vi "Sistema_Aquisicao_queued.vi"() -> ()   [LabVIEW 2018]
uses:
  Global_Telescopio.vi
panel:
  out "respQ":refnum<queue>
  out "cmdQ":refnum<queue>
  out "error out":errorcluster
  out "ultimo valor 2":dbl format="%#_9g"
  out "ultimo valor":dbl format="%#_9g"
  out "ultimo comando":dbl
  in  "Case Constant\n(See Context Help)":bool=TRUE
  out "O Recebido":bool
  out "TimeoutAq":u32
  out "concatenated string":string
  out "Maq Satus":i32
  out "TX":string
  out "Data rx Aquisição":string
  # "2"
  # "R -->Registra Centragem\nS -->Status\nO -->OffSet\nF ---> Foco"
  # "3"
  # "4"
  # "5"
  # "!"
  # "!"
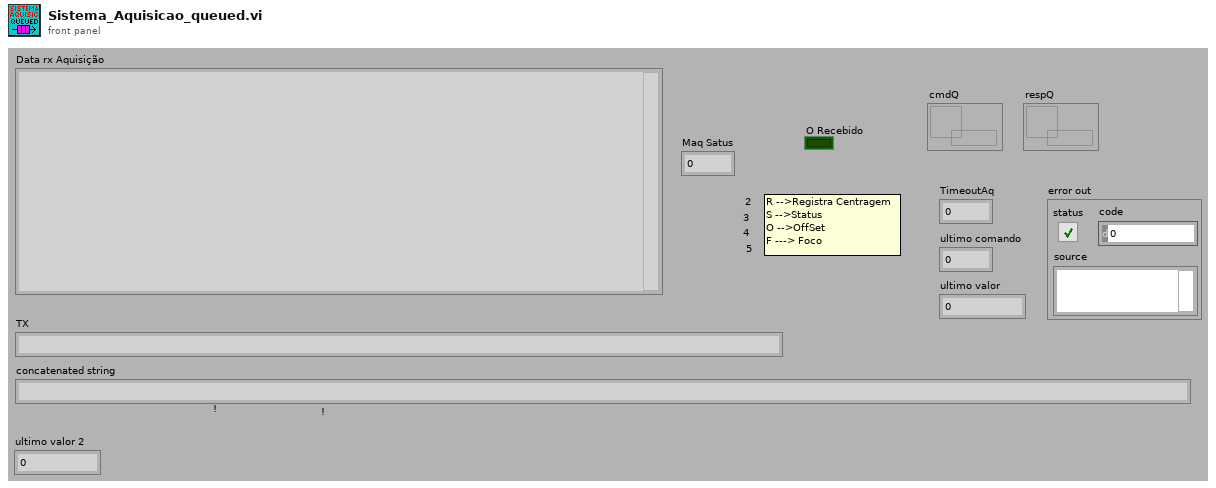
[diagram p1: front panel]
types:
  T1 = enum16{"open", "open or create", "create or replace", "create"}
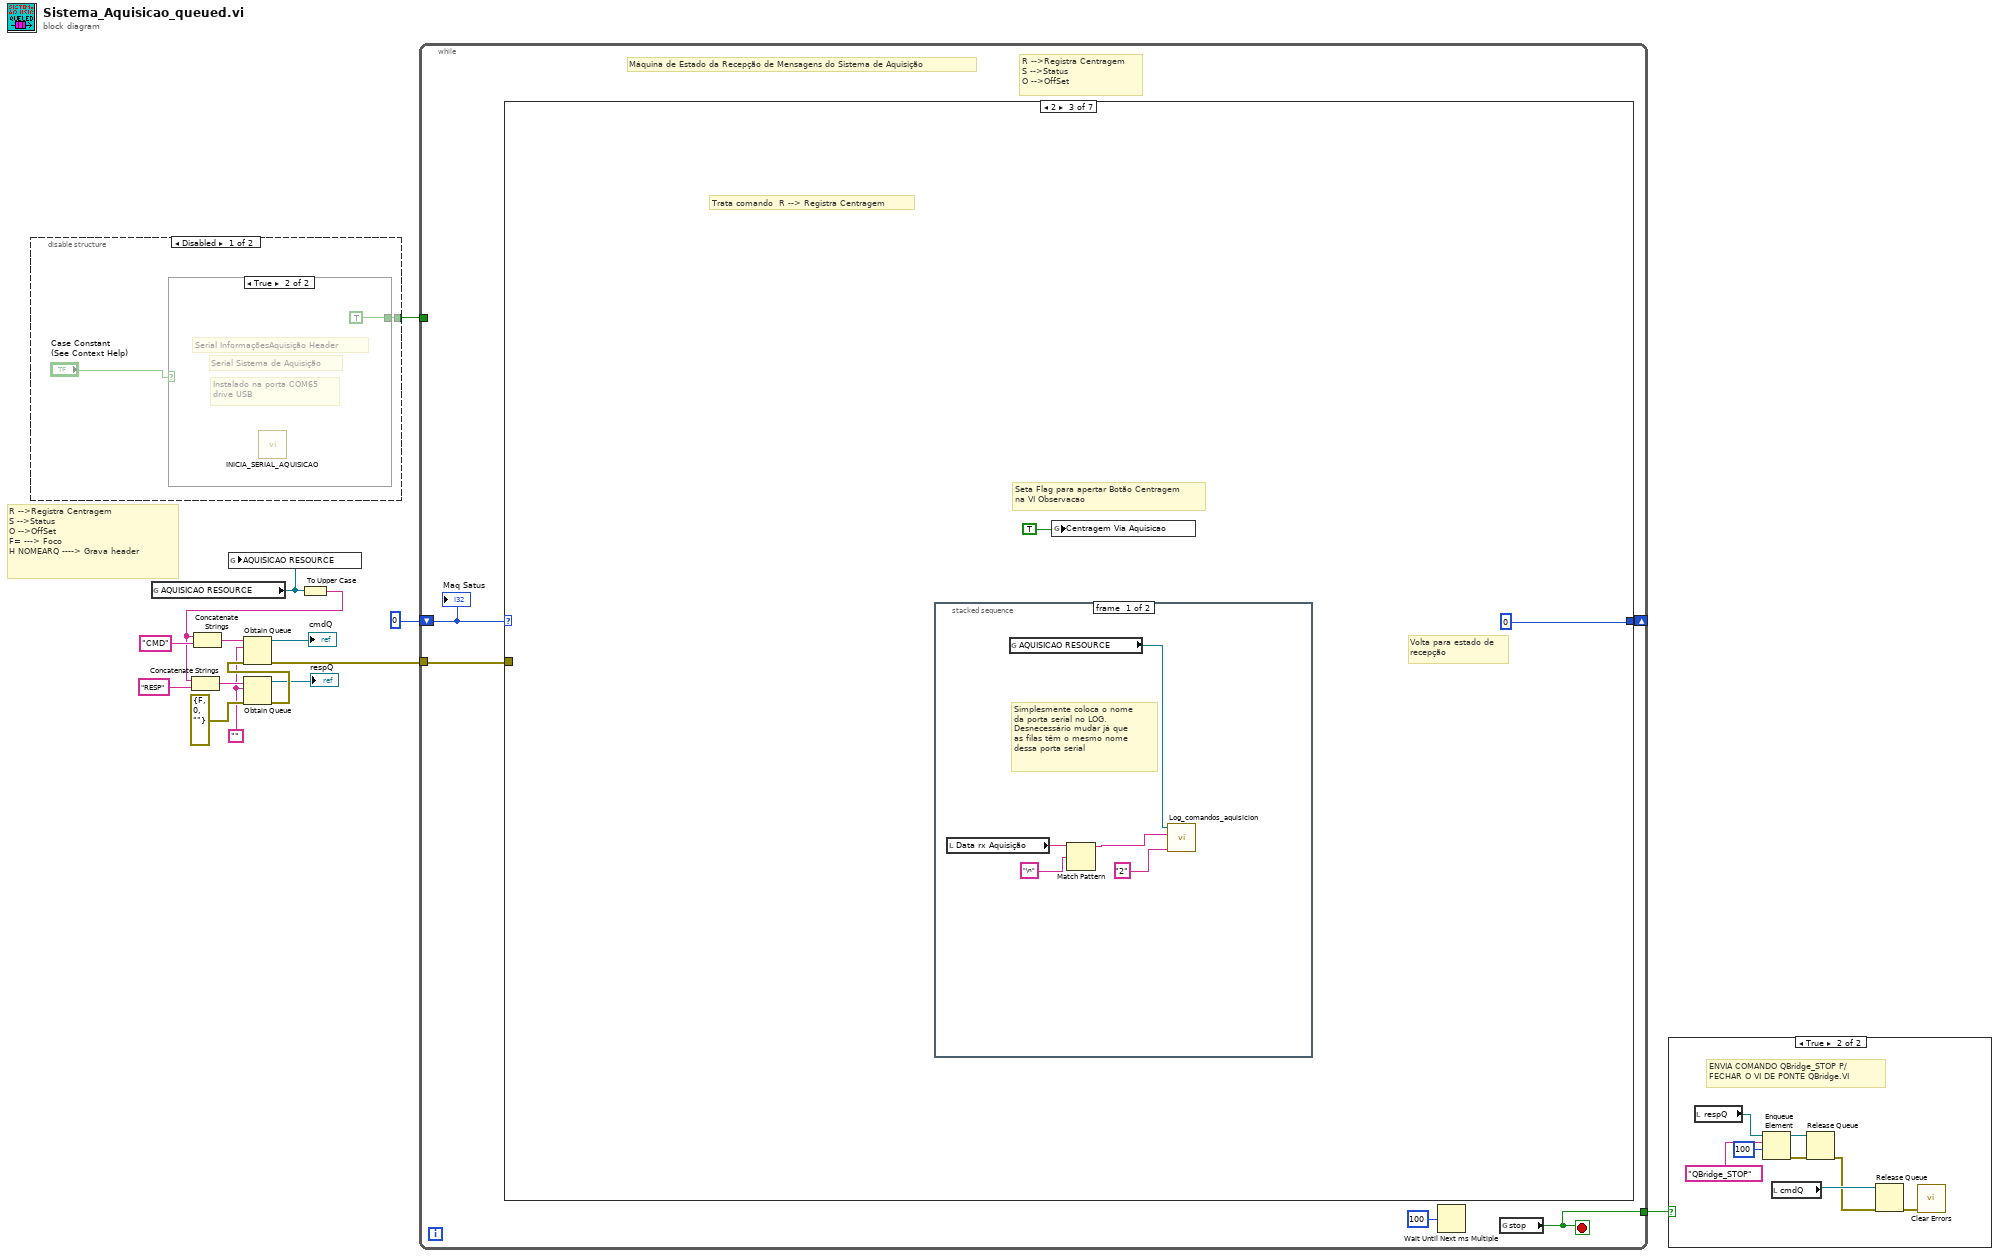
[diagram p0: block diagram]
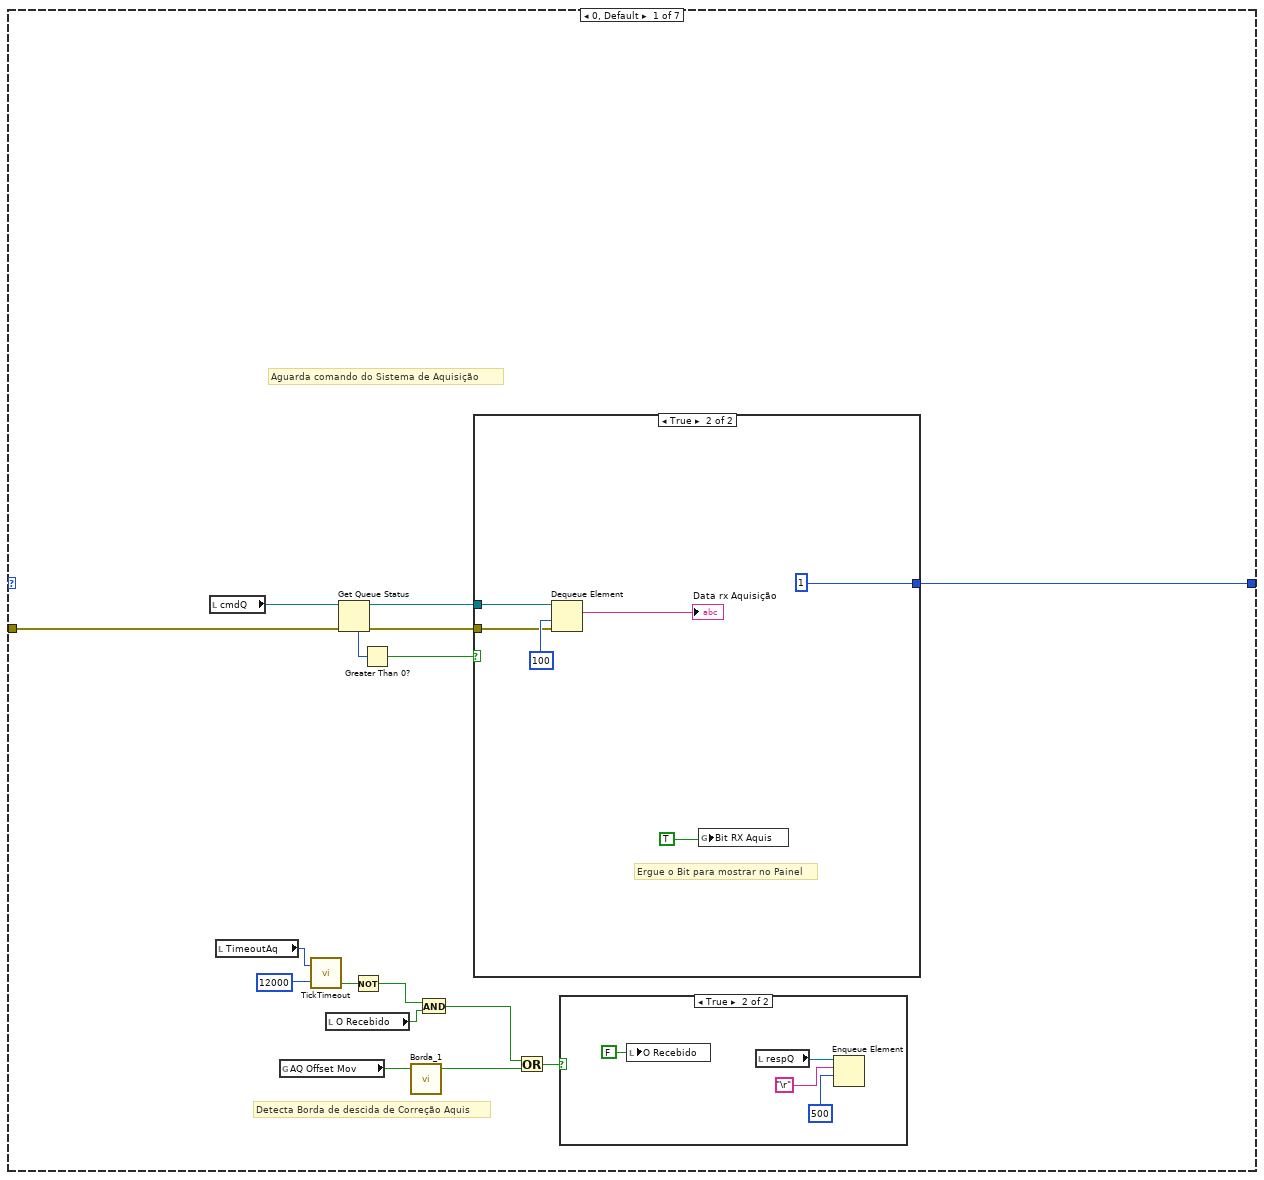
[diagram p5: hidden frame]
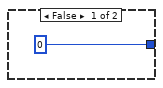
[diagram p7: hidden frame]
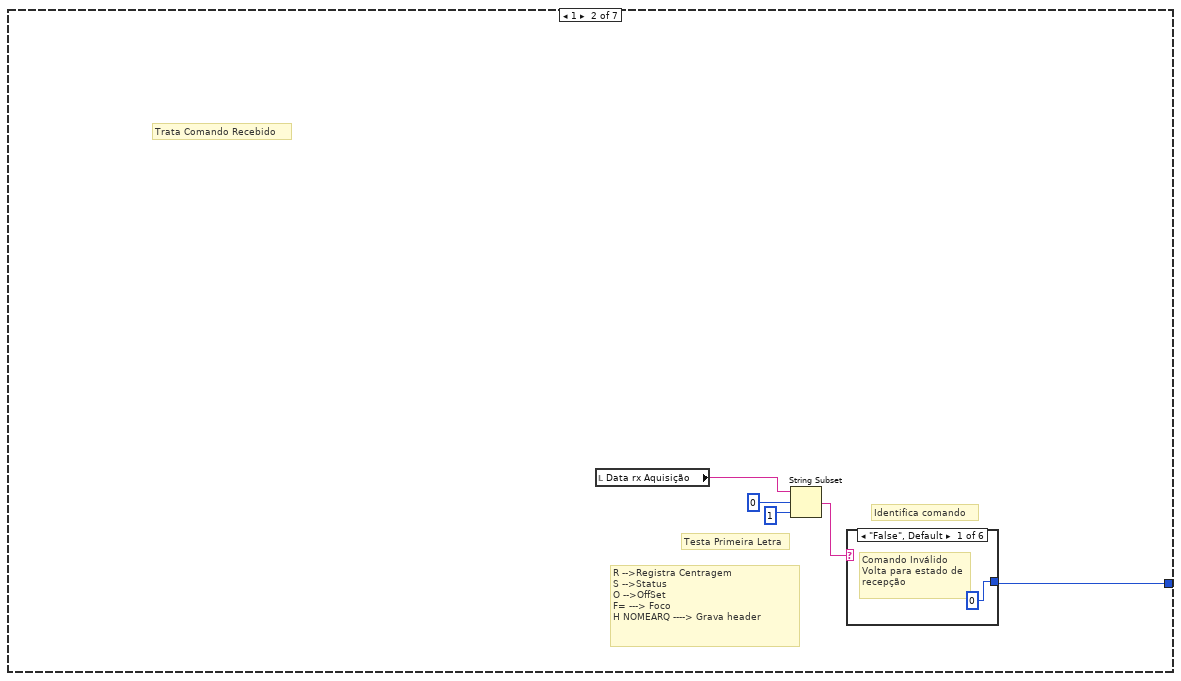
[diagram p8: hidden frame]
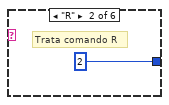
[diagram p9: hidden frame]
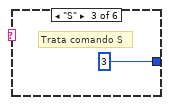
[diagram p10: hidden frame]
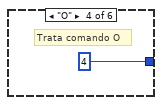
[diagram p11: hidden frame]
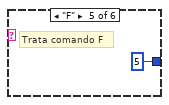
[diagram p12: hidden frame]
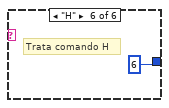
[diagram p13: hidden frame]
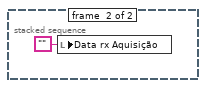
[diagram p14: hidden frame]
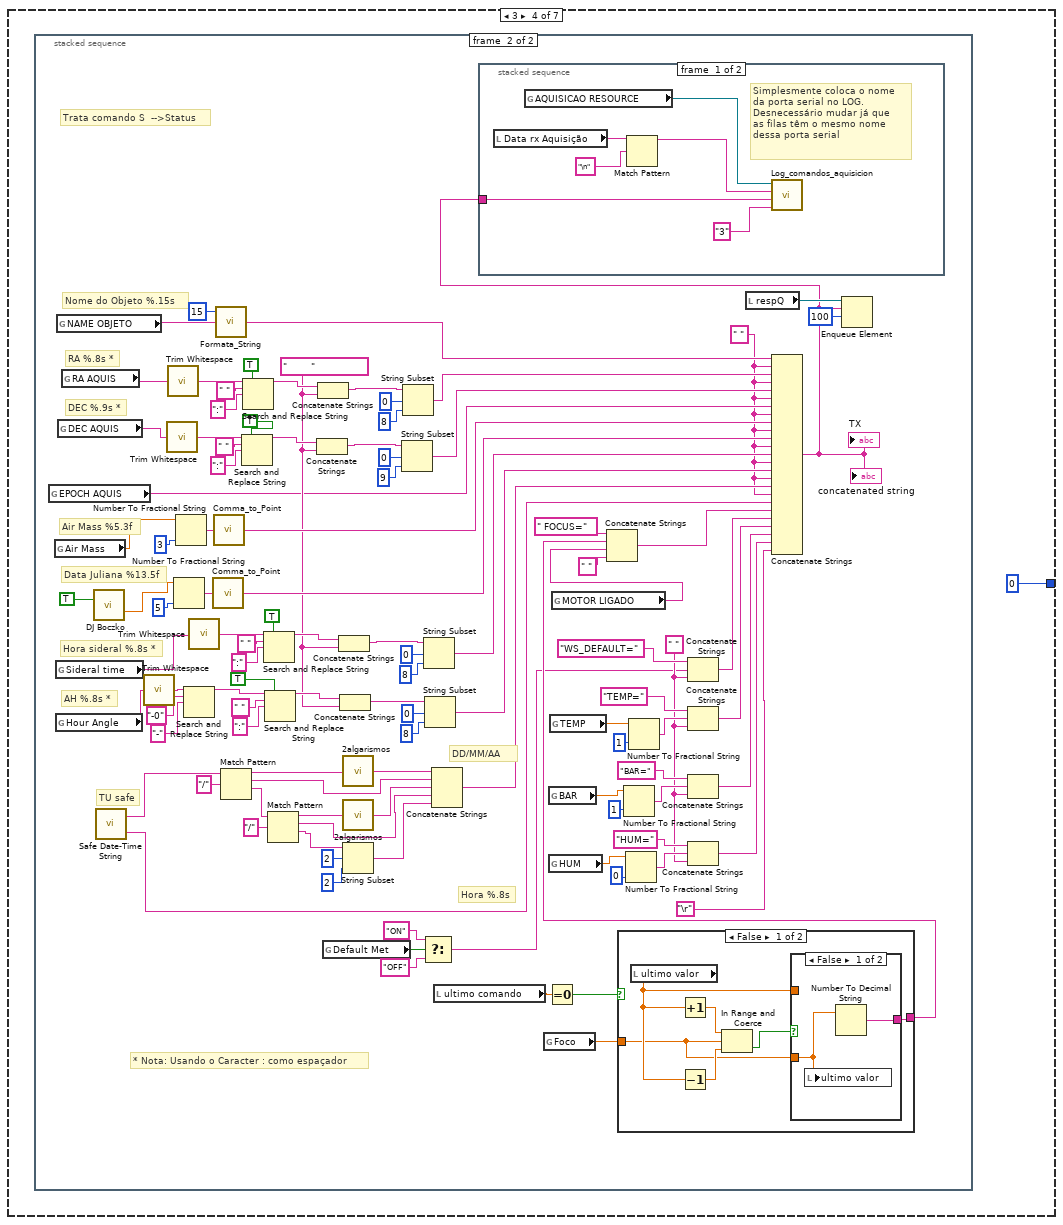
[diagram p15: hidden frame]
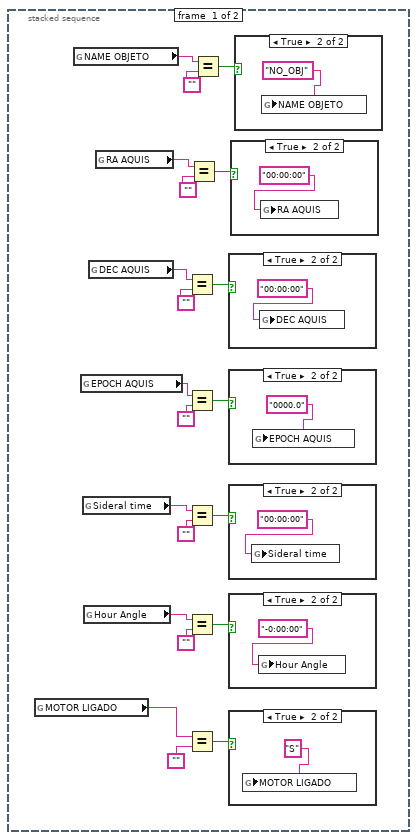
[diagram p16: hidden frame]
diagram:
  w5 = ""
  # "R -->Registra Centragem\nS -->Status\nO -->OffSet\nF= ---> Foco\nH NOMEARQ ----> Grava header"
  n1 = disable-structure shown="Disabled" {
    disable-tunnel: [w16 _] -> w14
    frame Disabled {
      n2 = case shown="True" "Case Constant\n(See Context Help)" {
        tunnel: [_ TRUE] -> w16
        frame False {
        }
        frame True {
          # "Instalado na porta COM65\ndrive USB"
          # "Serial Sistema de Aquisição"
          # "Serial InformaçõesAquisição Header"
          n3 = call "INICIA_SERIAL_AQUISICAO.vi"() -> ()  [unwired: 1 in]
        }
      }
    }
    frame Enabled {
    }
  }
  n4 = global read "Global_Telescopio.vi" "AQUISICAO RESOURCE"() -> (w3:refnum<visa-resource-name>)
  n5 = global write "Global_Telescopio.vi" "AQUISICAO RESOURCE"(w3) -> ()
  n6 = To Upper Case(1:w3) -> (0:w2:string)
  n7 = Concatenate Strings(w2, "RESP" ("string")) -> (w11:string)
  n8 = Concatenate Strings(w2, "CMD" ("string")) -> (w10:string)
  n9 = Obtain Queue(name (unnamed)=w11, element data type=w5, error in (no error)=errorcluster {"status"=FALSE, "code"=0, "source"=""}) -> (queue out=→"respQ":refnum<queue>, error out=w8:errorcluster)  [unwired: 2 in, 1 out]
  n10 = Obtain Queue(name (unnamed)=w10, element data type=w5, error in (no error)=w8) -> (queue out=→"cmdQ":refnum<queue>, error out=w4:errorcluster)  [unwired: 2 in, 1 out]
  n11 = while {
    shift-right: [w21] -> _
    shift-left: 0 -> [w22]
    tunnel: w14 -> [_]
    tunnel: w4 -> [w20]
    tunnel: [w19] -> w1
    stop <- w19 stop-if-true
    # "R -->Registra Centragem\nS -->Status\nO -->OffSet"
    # "Máquina de Estado da Recepção de Mensagens do Sistema de Aquisição"
    n12 = case shown="2" w22 {
      tunnel: [w39 w51 0 0 0 0 0] -> w21
      tunnel: w20 -> [w25 _ _ _ _ _ _]
      frame 0, Default {
        # "Detecta Borda de descida de Correção Aquis"
        # "Aguarda comando do Sistema de Aquisição"
        n13 = local read "cmdQ"() -> (w24:refnum<queue>)
        n14 = local read "TimeoutAq"() -> (w32:u32)
        n15 = global read "Global_Telescopio.vi" "AQ Offset Mov"() -> (w37:bool)
        n16 = call "TickTimeout.vi"("msInicial"=w32, "msTimeout"=u32 12000) -> ("Timeout"=w33:bool)  [unwired: 2 out]
        n17 = local read "O Recebido"() -> (w35:bool)
        n18 = Get Queue Status(queue=w24, error in (no error)=w25) -> (queue out=w26:refnum<queue>, error out=w27:errorcluster, # elements in queue=w29:i32)  [unwired: 1 in, 5 out]
        n19 = Not(x=w33) -> (.not. x?=w31:bool)
        n20 = Greater Than 0?(x=w29) -> (x > 0?=w28:bool)
        n21 = call "Borda_1.vi"("Entrada"=w37) -> ("Boolean"=w38:bool)  [unwired: 4 in]
        n22 = And(x=w31, y=w35) -> (x .and. y?=w30:bool)
        n23 = case shown="True" w28 {
          tunnel: [0 1] -> w39
          tunnel: w27 -> [_ w46]
          tunnel: w26 -> [_ w47]
          frame False {
          }
          frame True {
            # "Ergue o Bit para mostrar no Painel"
            n24 = Dequeue Element(queue=w47, timeout in ms (-1)=100, error in (no error)=w46) -> (element=→"Data rx Aquisição":string)  [unwired: 3 out]
            n25 = global write "Global_Telescopio.vi" "Bit RX Aquis"(TRUE) -> ()
          }
        }
        n26 = Or(x=w30, y=w38) -> (x .or. y?=w36:bool)
        n27 = case shown="True" w36 {
          frame False {
          }
          frame True {
            n28 = local write "O Recebido"(FALSE ("O Recebido")) -> ()
            n29 = local read "respQ"() -> (w42:refnum<queue>)
            n30 = Enqueue Element(queue=w42, element="\r", timeout in ms (-1)=500) -> ()  [unwired: 1 in, 3 out]
          }
        }
      }
      frame 1 {
        # "R -->Registra Centragem\nS -->Status\nO -->OffSet\nF= ---> Foco\nH NOMEARQ ----> Grava header"
        # "Testa Primeira Letra"
        # "Identifica comando"
        # "Trata Comando Recebido"
        n31 = local read "Data rx Aquisição"() -> (w52:string)
        n32 = String Subset(string=w52, offset (0)=0, length (rest)=1 ("length (rest)")) -> (substring=w55:string)
        n33 = case shown="\"False\", Default" w55 {
          tunnel: [0 2 3 4 5 6] -> w51
          frame "False", Default {
            # "Comando Inválido\nVolta para estado de\nrecepção"
          }
          frame "R" {
            # "Trata comando R"
          }
          frame "S" {
            # "Trata comando S"
          }
          frame "O" {
            # "Trata comando O"
          }
          frame "F" {
            # "Trata comando F"
          }
          frame "H" {
            # "Trata comando H"
          }
        }
      }
      frame 2 {
        # "Seta Flag para apertar Botão Centragem\nna VI Observacao"
        # "Trata comando  R --> Registra Centragem"
        # "Volta para estado de\nrecepção"
        n34 = stacked-sequence {
          frame #0 {
            # "Simplesmente coloca o nome\nda porta serial no LOG.\nDesnecessário mudar já que \nas filas têm o mesmo nome\ndessa porta serial"
            n35 = local read "Data rx Aquisição"() -> (w65:string)
            n36 = global read "Global_Telescopio.vi" "AQUISICAO RESOURCE"() -> (w68:refnum<visa-resource-name>)
            n37 = Match Pattern(string=w65, regular expression="\n") -> (before substring=w64:string)  [unwired: 1 in, 3 out]
            n38 = call "Log_comandos_aquisicion.vi"("Estado"="2", "string de comando"=w64, "Porta"=w68) -> ()  [unwired: 9 in]
          }
          frame #1 {
            n39 = local write "Data rx Aquisição"("") -> ()
          }
        }
        n40 = global write "Global_Telescopio.vi" "Centragem Via Aquisicao"(TRUE ("Comunicaçao ok guider")) -> ()
      }
      frame 3 {
        n41 = stacked-sequence {
          frame #0 {
            n42 = global read "Global_Telescopio.vi" "MOTOR LIGADO"() -> (w91:string)
            n43 = global read "Global_Telescopio.vi" "NAME OBJETO"() -> (w72:string)
            n44 = global read "Global_Telescopio.vi" "EPOCH AQUIS"() -> (w81:string)
            n45 = global read "Global_Telescopio.vi" "Sideral time"() -> (w83:string)
            n46 = global read "Global_Telescopio.vi" "Hour Angle"() -> (w88:string)
            n47 = global read "Global_Telescopio.vi" "DEC AQUIS"() -> (w79:string)
            n48 = global read "Global_Telescopio.vi" "RA AQUIS"() -> (w76:string)
            n49 = Equal?(x=w79, y="") -> (x = y?=w78:bool)
            n50 = Equal?(x=w81, y="") -> (x = y?=w80:bool)
            n51 = Equal?(x=w83, y="") -> (x = y?=w82:bool)
            n52 = Equal?(x=w88, y="") -> (x = y?=w84:bool)
            n53 = Equal?(x=w91, y="") -> (x = y?=w90:bool)
            n54 = Equal?(x=w76, y="") -> (x = y?=w74:bool)
            n55 = Equal?(x=w72, y="") -> (x = y?=w73:bool)
            n56 = case shown="True" w78 {
              frame False {
              }
              frame True {
                n57 = global write "Global_Telescopio.vi" "DEC AQUIS"("00:00:00" ("NAME OBJETO")) -> ()
              }
            }
            n58 = case shown="True" w80 {
              frame False {
              }
              frame True {
                n59 = global write "Global_Telescopio.vi" "EPOCH AQUIS"("0000.0" ("NAME OBJETO")) -> ()
              }
            }
            n60 = case shown="True" w82 {
              frame False {
              }
              frame True {
                n61 = global write "Global_Telescopio.vi" "Sideral time"("00:00:00" ("NAME OBJETO")) -> ()
              }
            }
            n62 = case shown="True" w84 {
              frame False {
              }
              frame True {
                n63 = global write "Global_Telescopio.vi" "Hour Angle"("-0:00:00" ("NAME OBJETO")) -> ()
              }
            }
            n64 = case shown="True" w90 {
              frame False {
              }
              frame True {
                n65 = global write "Global_Telescopio.vi" "MOTOR LIGADO"("S") -> ()
              }
            }
            n66 = case shown="True" w74 {
              frame False {
              }
              frame True {
                n67 = global write "Global_Telescopio.vi" "RA AQUIS"("00:00:00" ("NAME OBJETO")) -> ()
              }
            }
            n68 = case shown="True" w73 {
              frame False {
              }
              frame True {
                n69 = global write "Global_Telescopio.vi" "NAME OBJETO"("NO_OBJ" ("NAME OBJETO")) -> ()
              }
            }
          }
          frame #1 {
            w113 = " " ("string")
            w163 = "        " ("string")
            w121 = " "
            # "TU safe"
            # "* Nota: Usando o Caracter : como espaçador"
            # "Hora %.8s"
            # "DD/MM/AA"
            # "AH %.8s *"
            # "Hora sideral %.8s *"
            # "Data Juliana %13.5f"
            # "Air Mass %5.3f"
            # "DEC %.9s *"
            # "RA %.8s *"
            # "Nome do Objeto %.15s"
            # "Trata comando S  -->Status"
            n70 = global read "Global_Telescopio.vi" "EPOCH AQUIS"() -> (w136:string)
            n71 = global read "Global_Telescopio.vi" "Air Mass"() -> (w145:dbl)
            n72 = global read "Global_Telescopio.vi" "Sideral time"() -> (w172:string)
            n73 = global read "Global_Telescopio.vi" "Hour Angle"() -> (w137:string)
            n74 = global read "Global_Telescopio.vi" "NAME OBJETO"() -> (w144:string)
            n75 = global read "Global_Telescopio.vi" "DEC AQUIS"() -> (w189:string)
            n76 = global read "Global_Telescopio.vi" "RA AQUIS"() -> (w204:string)
            n77 = call "DJ Boczko.vi"("TRUE = Hora Local\nFALSE = UT"=TRUE ("TRUE = Hora Local\nFALSE = UT")) -> ("Dia Juliano"=w182:dbl)  [unwired: 6 in, 8 out]
            n78 = call "Safe Date-Time String.vi"() -> ("Safe time string"=w100:string, "Safe date string"=w99:string)  [unwired: 3 in]
            n79 = call <vilib>:"Trim Whitespace.vi"("string"=w137) -> ("trimmed string"=w138:string)  [unwired: 1 in]
            n80 = call <vilib>:"Trim Whitespace.vi"("string"=w189) -> ("trimmed string"=w192:string)  [unwired: 1 in]
            n81 = call <vilib>:"Trim Whitespace.vi"("string"=w204) -> ("trimmed string"=w203:string)  [unwired: 1 in]
            n82 = Number To Fractional String(number=w182, precision (6)=i16 5) -> (F-format string=w181:string)  [unwired: 2 in]
            n83 = Number To Fractional String(number=w145, precision (6)=i16 3) -> (F-format string=w185:string)  [unwired: 2 in]
            n84 = Search and Replace String(input string=w138, search string="-0", replace string="-" ("replace string (\"\")")) -> (result string=w139:string)  [unwired: 5 in, 3 out]
            n85 = call <vilib>:"Trim Whitespace.vi"("string"=w172) -> ("trimmed string"=w175:string)  [unwired: 1 in]
            n86 = call "Comma_to_Point.vi"("Lat_A"=w181) -> ("Saída"=w180:string)
            n87 = call "Comma_to_Point.vi"("Lat_A"=w185) -> ("Saída"=w184:string)
            n88 = call "Formata_String.vi"("entrada"=w144, "Num de Caracteres"=15) -> ("saida"=w142:string)  [unwired: 3 in]
            n89 = Match Pattern(string=w99, regular expression="/") -> (before substring=w158:string, match substring=w152:string, after substring=w159:string)  [unwired: 1 in, 1 out]
            n90 = Search and Replace String(replace all?=TRUE ("replace all? (F)"), input string=w192, search string=" ", replace string=":" ("replace string (\"\")")) -> (result string=w195:string)  [unwired: 4 in, 3 out]
            n91 = Search and Replace String(replace all?=TRUE ("replace all? (F)"), input string=w203, search string=" ", replace string=":" ("replace string (\"\")")) -> (result string=w199:string)  [unwired: 4 in, 3 out]
            n92 = Search and Replace String(replace all?=TRUE ("replace all? (F)"), input string=w175, search string=" ", replace string=":" ("replace string (\"\")")) -> (result string=w178:string)  [unwired: 4 in, 3 out]
            n93 = Search and Replace String(replace all?=TRUE ("replace all? (F)"), input string=w139, search string=" ", replace string=":" ("replace string (\"\")")) -> (result string=w165:string)  [unwired: 4 in, 3 out]
            n94 = Match Pattern(string=w159, regular expression="/") -> (before substring=w157:string, match substring=w150:string, after substring=w156:string)  [unwired: 1 in, 1 out]
            n95 = Concatenate Strings(w195, w163) -> (w196:string)
            n96 = Concatenate Strings(w199, w163) -> (w198:string)
            n97 = global read "Global_Telescopio.vi" "Default Met"() -> (w104:bool)
            n98 = Concatenate Strings(w178, w163) -> (w179:string)
            n99 = Concatenate Strings(w165, w163) -> (w164:string)
            n100 = call "2algarismos.vi"("entrada"=w158) -> ("saida"=w153:string)
            n101 = call "2algarismos.vi"("entrada"=w157) -> ("saida"=w151:string)
            n102 = String Subset(string=w156, offset (0)=2, length (rest)=2 ("length (rest)")) -> (substring=w149:string)
            n103 = String Subset(string=w196, offset (0)=0, length (rest)=9 ("length (rest)")) -> (substring=w188:string)
            n104 = String Subset(string=w198, offset (0)=0, length (rest)=8 ("length (rest)")) -> (substring=w197:string)
            n105 = Select(t="ON", s=w104, f="OFF") -> (s? t:f=w101:string)
            n106 = String Subset(string=w179, offset (0)=0, length (rest)=8 ("length (rest)")) -> (substring=w170:string)
            n107 = String Subset(string=w164, offset (0)=0, length (rest)=8 ("length (rest)")) -> (substring=w162:string)
            n108 = Concatenate Strings(w153, w152, w151, w150, w149) -> (w148:string)
            n109 = local read "ultimo comando"() -> (w135:dbl)
            n110 = global read "Global_Telescopio.vi" "Foco"() -> (w130:dbl)
            n111 = Equal To 0?(x=w135) -> (x = 0?=w134:bool)
            n112 = global read "Global_Telescopio.vi" "BAR"() -> (w123:dbl)
            n113 = global read "Global_Telescopio.vi" "HUM"() -> (w122:dbl)
            n114 = global read "Global_Telescopio.vi" "TEMP"() -> (w127:dbl)
            n115 = global read "Global_Telescopio.vi" "MOTOR LIGADO"() -> (w129:string)
            n116 = case shown="False" w134 {
              tunnel: [w215 w225] -> w133
              tunnel: w130 -> [w214 w224]
              frame False {
                n117 = local read "ultimo valor"() -> (w216:dbl)
                n118 = Increment(x=w216) -> (x+1=w218:dbl)
                n119 = Decrement(x=w216) -> (x-1=w217:dbl)
                n120 = In Range and Coerce(upper limit=w218, x=w214, lower limit=w217) -> (In Range?=w219:bool)  [unwired: 1 out]
                n121 = case shown="False" w219 {
                  tunnel: w216 -> [_ w223]
                  tunnel: [w221 w222] -> w215
                  tunnel: w214 -> [w220 _]
                  frame False {
                    n122 = local write "ultimo valor"(w220) -> ()
                    n123 = Number To Decimal String(number=w220) -> (decimal integer string=w221:string)  [unwired: 1 in]
                  }
                  frame True {
                    n124 = Number To Decimal String(number=w223) -> (decimal integer string=w222:string)  [unwired: 1 in]
                  }
                }
              }
              frame True {
                n125 = Number To Decimal String(number=w224) -> (decimal integer string=w225:string)  [unwired: 1 in]
                "ultimo valor" <- w224
              }
            }
            n126 = Concatenate Strings(" FOCUS=" ("string"), w133, w129, " " ("string")) -> (w131:string)
            n127 = Number To Fractional String(number=w123, precision (6)=i16 1) -> (F-format string=w115:string)  [unwired: 2 in]
            n128 = Number To Fractional String(number=w122, precision (6)=i16 0) -> (F-format string=w114:string)  [unwired: 2 in]
            n129 = Number To Fractional String(number=w127, precision (6)=i16 1) -> (F-format string=w117:string)  [unwired: 2 in]
            n130 = Concatenate Strings("WS_DEFAULT=" ("string"), w101, w113) -> (w112:string)
            n131 = Concatenate Strings("TEMP=" ("string"), w117, w113) -> (w111:string)
            n132 = Concatenate Strings("BAR=" ("string"), w115, w113) -> (w110:string)
            n133 = Concatenate Strings("HUM=" ("string"), w114, w113) -> (w109:string)
            n134 = local read "respQ"() -> (w107:refnum<queue>)
            n135 = Concatenate Strings(w142, w121, w197, w121, w188, w121, w136, w121, w184, w121, w180, w121, w170, w121, w162, w121, w148, w121, w100, w131, w112, w111, w110, w109, "\r") -> (w106:string)
            "TX" <- w106
            "concatenated string" <- w106
            n136 = stacked-sequence {
              tunnel: w106 -> [w210 _]
              frame #0 {
                # "Simplesmente coloca o nome\nda porta serial no LOG.\nDesnecessário mudar já que \nas filas têm o mesmo nome\ndessa porta serial"
                n137 = local read "Data rx Aquisição"() -> (w209:string)
                n138 = global read "Global_Telescopio.vi" "AQUISICAO RESOURCE"() -> (w212:refnum<visa-resource-name>)
                n139 = Match Pattern(string=w209, regular expression="\n") -> (before substring=w207:string)  [unwired: 1 in, 3 out]
                n140 = call "Log_comandos_aquisicion.vi"("Estado"="3", "string de Resposta"=w210, "string de comando"=w207, "Porta"=w212) -> ()  [unwired: 8 in]
              }
              frame #1 {
                n141 = local write "Data rx Aquisição"("") -> ()
              }
            }
            n142 = Enqueue Element(queue=w107, element=w106, timeout in ms (-1)=100) -> ()  [unwired: 1 in, 3 out]
          }
        }
      }
      frame 4 {
        # "Trata comando O  -->OffSet"
        n143 = local read "Data rx Aquisição"() -> (w228:string)
        n144 = String Subset(string=w228, offset (0)=2, length (rest)=1 ("length (rest)")) -> (substring=w237:string)
        n145 = String Subset(string=w228, offset (0)=3, length (rest)=4 ("length (rest)")) -> (substring=w244:string)
        n146 = String Subset(string=w228, offset (0)=8, length (rest)=1 ("length (rest)")) -> (substring=w236:string)
        n147 = String Subset(string=w228, offset (0)=1, length (rest)=1 ("length (rest)")) -> (substring=w230:string)
        n148 = String Subset(string=w228, offset (0)=9, length (rest)=4 ("length (rest)")) -> (substring=w243:string)
        n149 = Fract/Exp String To Number(use system decimal point (T)=FALSE, string=w244) -> (number=w233:dbl)  [unwired: 2 in, 1 out]
        n150 = Fract/Exp String To Number(use system decimal point (T)=FALSE, string=w243) -> (number=w231:dbl)  [unwired: 2 in, 1 out]
        n151 = case shown="\"N\"" w237 {
          tunnel: [0.0 ("PreciseOffsetDEC 2") 1.0 ("PreciseOffsetDEC 2") -1.0 ("PreciseOffsetDEC 2")] -> w234
          frame " ", Default {
          }
          frame "N" {
          }
          frame "S" {
          }
        }
        n152 = case shown="\"E\"" w236 {
          tunnel: [0.0 ("PreciseOffsetDEC 2") 1.0 ("PreciseOffsetDEC 2") -1.0 ("PreciseOffsetDEC 2")] -> w232
          frame " ", Default {
          }
          frame "W" {
          }
          frame "E" {
          }
        }
        n153 = call "Salva_comando_Apend.vi"("String"=w228, "file name p/ exell"="C:\\TCS\\LOG\\Comando_O_Aquisicao.txt") -> ()  [unwired: 4 in]
        n154 = Multiply(x=w234, y=w232) -> (x*y=w238:dbl)
        n155 = Equal To 0?(x=w238) -> (x = 0?=w235:bool)
        n156 = case shown="True" w235 {
          tunnel: w234 -> [w271 _]
          tunnel: w233 -> [w270 _]
          tunnel: w232 -> [w269 _]
          tunnel: w231 -> [w268 _]
          tunnel: w230 -> [w266 _]
          tunnel: [TRUE ("Correção Aquis") FALSE ("Correção Aquis")] -> w229
          tunnel: ["" ""] -> w226
          frame False {
            n157 = Multiply(x=w271, y=w270) -> (x*y=w263:dbl)
            n158 = Multiply(x=w269, y=w268) -> (x*y=w267:dbl)
            n159 = case shown="\"1\"" w266 {
              tunnel: [1.0 ("PreciseOffsetDEC 2") w273] -> w265
              frame "0", Default {
              }
              frame "1" {
                n160 = global read "Global_Telescopio.vi" "delta_now"() -> (w274:dbl)
                n161 = Cosine(x=w274) -> (cos(x)=w275:dbl)
                n162 = Absolute Value(x=w275) -> (abs(x)=w273:dbl)
              }
            }
            n163 = Divide(x=w267, y=w265) -> (x/y=w264:dbl)
            n164 = global write "Global_Telescopio.vi" "aquis_asc"(w264) -> ()
            n165 = global write "Global_Telescopio.vi" "aquis_dec"(w263) -> ()
            n166 = call "TickTimeout.vi"() -> ("msTick"=→"TimeoutAq":u32)  [unwired: 2 in, 2 out]
          }
          frame True {
          }
        }
        "O Recebido" <- w229
        n167 = stacked-sequence {
          tunnel: w226 -> [_ w259]
          frame #0 {
            n168 = local read "Data rx Aquisição"() -> (w255:string)
            n169 = global read "Global_Telescopio.vi" "AQUISICAO RESOURCE"() -> (w258:refnum<visa-resource-name>)
            n170 = Match Pattern(string=w255, regular expression="\n") -> (before substring=w254:string)  [unwired: 1 in, 3 out]
            n171 = call "Log_comandos_aquisicion.vi"("Estado"="4", "string de comando"=w254, "Porta"=w258) -> ()  [unwired: 9 in]
          }
          frame #1 {
            n172 = local write "Data rx Aquisição"(w259) -> ()
          }
        }
        n173 = global write "Global_Telescopio.vi" "Correção Aquis"(w229) -> ()
      }
      frame 5 {
        # "Trata comando F ---> Trata o comando de foco vindo do computador de aquisição"
        n174 = local read "Data rx Aquisição"() -> (w292:string)
        n175 = Match Pattern(string=w292, regular expression="=") -> (after substring=w290:string)  [unwired: 1 in, 3 out]
        n176 = Fract/Exp String To Number(string=w290) -> (number=w286:dbl)  [unwired: 3 in, 1 out]
        n177 = In Range and Coerce(upper limit=2012.0, x=w286, lower limit=1.0) -> (In Range?=w287:bool)  [unwired: 1 out]
        n178 = case shown="True" w287 {
          tunnel: w286 -> [_ w302]
          tunnel: ["" ""] -> w284
          frame False {
          }
          frame True {
            n179 = case shown="True" TRUE {
              tunnel: ["stop" ("Comando") "go" ("Comando")] -> w301
              frame False {
              }
              frame True {
                n180 = call "TX focus FOCO.vi"("Comando"="def", "Setpoint"=20.0) -> ()  [unwired: 11 in, 3 out]
              }
            }
            n181 = call "TX focus FOCO.vi"("Comando"=w301, "Setpoint"=w302) -> ()  [unwired: 11 in, 3 out]
            "ultimo comando" <- w302
          }
        }
        n182 = stacked-sequence {
          tunnel: w284 -> [_ w298]
          frame #0 {
            n183 = local read "Data rx Aquisição"() -> (w294:string)
            n184 = global read "Global_Telescopio.vi" "AQUISICAO RESOURCE"() -> (w297:refnum<visa-resource-name>)
            n185 = Match Pattern(string=w294, regular expression="\n") -> (before substring=w293:string)  [unwired: 1 in, 3 out]
            n186 = call "Log_comandos_aquisicion.vi"("Estado"="5", "string de comando"=w293, "Porta"=w297) -> ()  [unwired: 9 in]
          }
          frame #1 {
            n187 = local write "Data rx Aquisição"(w298) -> ()
          }
        }
      }
      frame 6 {
        w338 = " " ("string")
        w388 = "        " ("string")
        w346 = " "
        # "TU safe"
        # "ANTES DE INTRODUZIR FILAS\nESTA ESTRUTURA DISABLE JÁ\nESTAVA PRESENTE NO CÓDIGO"
        # "file name"
        # "* Nota: Usando o Caracter : como espaçador"
        # "Hora %.8s"
        # "DD/MM/AA"
        # "AH %.8s *"
        # "Hora sideral %.8s *"
        # "Data Juliana %13.5f"
        # "Air Mass %5.3f"
        # "DEC %.9s *"
        # "RA %.8s *"
        # "Nome do Objeto %.15s"
        # "Trata comando H NOMEARQ ---> Grava Header"
        n188 = global read "Global_Telescopio.vi" "EPOCH AQUIS"() -> (w361:string)
        n189 = global read "Global_Telescopio.vi" "Air Mass"() -> (w370:dbl)
        n190 = global read "Global_Telescopio.vi" "Sideral time"() -> (w397:string)
        n191 = global read "Global_Telescopio.vi" "Hour Angle"() -> (w362:string)
        n192 = global read "Global_Telescopio.vi" "NAME OBJETO"() -> (w369:string)
        n193 = global read "Global_Telescopio.vi" "DEC AQUIS"() -> (w414:string)
        n194 = global read "Global_Telescopio.vi" "RA AQUIS"() -> (w429:string)
        n195 = call "DJ Boczko.vi"("TRUE = Hora Local\nFALSE = UT"=TRUE ("TRUE = Hora Local\nFALSE = UT")) -> ("Dia Juliano"=w407:dbl)  [unwired: 6 in, 8 out]
        n196 = call "Safe Date-Time String.vi"() -> ("Safe time string"=w309:string, "Safe date string"=w308:string)  [unwired: 3 in]
        n197 = call <vilib>:"Trim Whitespace.vi"("string"=w362) -> ("trimmed string"=w363:string)  [unwired: 1 in]
        n198 = local read "Data rx Aquisição"() -> (w332:string)
        n199 = call <vilib>:"Trim Whitespace.vi"("string"=w414) -> ("trimmed string"=w417:string)  [unwired: 1 in]
        n200 = call <vilib>:"Trim Whitespace.vi"("string"=w429) -> ("trimmed string"=w428:string)  [unwired: 1 in]
        n201 = Number To Fractional String(number=w407, precision (6)=i16 5) -> (F-format string=w406:string)  [unwired: 2 in]
        n202 = Number To Fractional String(number=w370, precision (6)=i16 3) -> (F-format string=w410:string)  [unwired: 2 in]
        n203 = Search and Replace String(input string=w363, search string="-0", replace string="-" ("replace string (\"\")")) -> (result string=w364:string)  [unwired: 5 in, 3 out]
        n204 = call <vilib>:"Trim Whitespace.vi"("string"=w397) -> ("trimmed string"=w400:string)  [unwired: 1 in]
        n205 = Match Pattern(string=w332, regular expression="H ") -> (after substring=w317:string)  [unwired: 1 in, 3 out]
        n206 = call "Comma_to_Point.vi"("Lat_A"=w406) -> ("Saída"=w405:string)
        n207 = call "Comma_to_Point.vi"("Lat_A"=w410) -> ("Saída"=w409:string)
        n208 = call "Formata_String.vi"("entrada"=w369, "Num de Caracteres"=15) -> ("saida"=w367:string)  [unwired: 3 in]
        n209 = Match Pattern(string=w308, regular expression="/") -> (before substring=w383:string, match substring=w377:string, after substring=w384:string)  [unwired: 1 in, 1 out]
        n210 = global read "Global_Telescopio.vi" "Default Met"() -> (w313:bool)
        n211 = Search and Replace String(replace all?=TRUE ("replace all? (F)"), input string=w417, search string=" ", replace string=":" ("replace string (\"\")")) -> (result string=w420:string)  [unwired: 4 in, 3 out]
        n212 = Search and Replace String(replace all?=TRUE ("replace all? (F)"), input string=w428, search string=" ", replace string=":" ("replace string (\"\")")) -> (result string=w424:string)  [unwired: 4 in, 3 out]
        n213 = Search and Replace String(replace all?=TRUE ("replace all? (F)"), input string=w400, search string=" ", replace string=":" ("replace string (\"\")")) -> (result string=w403:string)  [unwired: 4 in, 3 out]
        n214 = Search and Replace String(replace all?=TRUE ("replace all? (F)"), input string=w364, search string=" ", replace string=":" ("replace string (\"\")")) -> (result string=w390:string)  [unwired: 4 in, 3 out]
        n215 = Match Pattern(string=w384, regular expression="/") -> (before substring=w382:string, match substring=w375:string, after substring=w381:string)  [unwired: 1 in, 1 out]
        n216 = Match Pattern(string=w317, regular expression="\r\n") -> (before substring=w315:string)  [unwired: 1 in, 3 out]
        n217 = Concatenate Strings(w420, w388) -> (w421:string)
        n218 = Concatenate Strings(w424, w388) -> (w423:string)
        n219 = Select(t="ON", s=w313, f="OFF") -> (s? t:f=w310:string)
        n220 = Concatenate Strings(w403, w388) -> (w404:string)
        n221 = Concatenate Strings(w390, w388) -> (w389:string)
        n222 = call "2algarismos.vi"("entrada"=w383) -> ("saida"=w378:string)
        n223 = call "2algarismos.vi"("entrada"=w382) -> ("saida"=w376:string)
        n224 = String Subset(string=w381, offset (0)=2, length (rest)=2 ("length (rest)")) -> (substring=w374:string)
        n225 = String Subset(string=w421, offset (0)=0, length (rest)=9 ("length (rest)")) -> (substring=w413:string)
        n226 = String Subset(string=w423, offset (0)=0, length (rest)=8 ("length (rest)")) -> (substring=w422:string)
        n227 = String Subset(string=w404, offset (0)=0, length (rest)=8 ("length (rest)")) -> (substring=w395:string)
        n228 = String Subset(string=w389, offset (0)=0, length (rest)=8 ("length (rest)")) -> (substring=w387:string)
        n229 = Concatenate Strings(w378, w377, w376, w375, w374) -> (w373:string)
        n230 = local read "ultimo comando"() -> (w360:dbl)
        n231 = global read "Global_Telescopio.vi" "Foco"() -> (w355:dbl)
        n232 = Equal To 0?(x=w360) -> (x = 0?=w359:bool)
        n233 = global read "Global_Telescopio.vi" "BAR"() -> (w348:dbl)
        n234 = global read "Global_Telescopio.vi" "HUM"() -> (w347:dbl)
        n235 = global read "Global_Telescopio.vi" "TEMP"() -> (w352:dbl)
        n236 = global read "Global_Telescopio.vi" "MOTOR LIGADO"() -> (w354:string)
        n237 = Concatenate Strings("C:\\TCS\\LOG\\HEADER\\" ("string"), w315, ".txt" ("string")) -> (w322:string)
        n238 = case shown="False" w359 {
          tunnel: [w436 w446] -> w358
          tunnel: w355 -> [w435 w445]
          frame False {
            n239 = local read "ultimo valor 2"() -> (w437:dbl)
            n240 = Increment(x=w437) -> (x+1=w439:dbl)
            n241 = Decrement(x=w437) -> (x-1=w438:dbl)
            n242 = In Range and Coerce(upper limit=w439, x=w435, lower limit=w438) -> (In Range?=w440:bool)  [unwired: 1 out]
            n243 = case shown="False" w440 {
              tunnel: w437 -> [_ w444]
              tunnel: [w442 w443] -> w436
              tunnel: w435 -> [w441 _]
              frame False {
                n244 = local write "ultimo valor 2"(w441) -> ()
                n245 = Number To Decimal String(number=w441) -> (decimal integer string=w442:string)  [unwired: 1 in]
              }
              frame True {
                n246 = Number To Decimal String(number=w444) -> (decimal integer string=w443:string)  [unwired: 1 in]
              }
            }
          }
          frame True {
            n247 = Number To Decimal String(number=w445) -> (decimal integer string=w446:string)  [unwired: 1 in]
            "ultimo valor 2" <- w445
          }
        }
        n248 = Concatenate Strings(" FOCUS=" ("string"), w358, w354, " " ("string")) -> (w356:string)
        n249 = Number To Fractional String(number=w348, precision (6)=i16 1) -> (F-format string=w340:string)  [unwired: 2 in]
        n250 = Number To Fractional String(number=w347, precision (6)=i16 0) -> (F-format string=w339:string)  [unwired: 2 in]
        n251 = Number To Fractional String(number=w352, precision (6)=i16 1) -> (F-format string=w342:string)  [unwired: 2 in]
        n252 = String To Path(string=w322) -> (path=w320:path)
        n253 = call <vilib>:"Open_Create_Replace File.vi"("function (open:0)"=T1."open or create", "file path"=w320) -> ("error out"=w327:errorcluster, "refnum"=w330:refnum<file>)  [unwired: 6 in, 2 out]
        n254 = Concatenate Strings("WS_DEFAULT=" ("string"), w310, w338) -> (w337:string)
        n255 = Concatenate Strings("TEMP=" ("string"), w342, w338) -> (w336:string)
        n256 = Concatenate Strings("BAR=" ("string"), w340, w338) -> (w335:string)
        n257 = Concatenate Strings("HUM=" ("string"), w339, w338) -> (w334:string)
        n258 = Set File Position(refnum=w330, from (0:start)=enum16{"start", "end", "current"}."end" ("pos mode (0:2)"), error in=w327) -> (refnum out=w324:refnum<file>, error out=w323:errorcluster)  [unwired: 1 in]
        n259 = Concatenate Strings(w367, w346, w422, w346, w413, w346, w361, w346, w409, w346, w405, w346, w395, w346, w387, w346, w373, w346, w309, w356, w337, w336, w335, w334, "\r") -> (w319:string)
        n260 = disable-structure shown="Disabled" {
          disable-tunnel: w319 -> [w433 _]
          frame Disabled {
            n261 = global read "Global_Telescopio.vi" "AQUISICAO RESOURCE"() -> (w434:refnum<visa-resource-name>)
            n262 = call "TX.vi"("tx_buf"=w433, "VISA resource name"=w434) -> ()  [unwired: 1 in, 3 out]
          }
          frame Enabled {
          }
        }
        n263 = Write to Text File(file (use dialog)=w324, text=w319, error in=w323) -> (refnum out=w329:refnum<file>, error out=w328:errorcluster)  [unwired: 1 in, 1 out]
        n264 = Close File(refnum=w329, error in=w328) -> (error out=→"error out":errorcluster)  [unwired: 1 out]
      }
    }
    n265 = Wait Until Next ms Multiple(millisecond multiple=u32 100) -> ()  [unwired: 1 out]
    n266 = global read "Global_Telescopio.vi" "stop"() -> (w19:bool)
    "Maq Satus" <- w22
  }
  n267 = case shown="True" w1 {
    frame False {
    }
    frame True {
      # "ENVIA COMANDO QBridge_STOP P/\nFECHAR O VI DE PONTE QBridge.VI"
      n268 = local read "respQ"() -> (w454:refnum<queue>)
      n269 = Enqueue Element(queue=w454, element="QBridge_STOP" ("x"), timeout in ms (-1)=100) -> (queue out=w453:refnum<queue>, error out=w452:errorcluster)  [unwired: 1 in, 1 out]
      n270 = local read "cmdQ"() -> (w451:refnum<queue>)
      n271 = Release Queue(queue=w453, error in (no error)=w452) -> (error out=w450:errorcluster)  [unwired: 1 in, 2 out]
      n272 = Release Queue(queue=w451, error in (no error)=w450) -> (error out=w448:errorcluster)  [unwired: 1 in, 2 out]
      n273 = call <vilib>:"Clear Errors.vi"("error in (no error)"=w448) -> ()  [unwired: 5 in, 2 out]
    }
  }
